vi "READ NavX.vi"() -> (1 "Status":T3 {"OP Status" items=["INITIALIZING", "SELFTEST_IN_PROGRESS", "ERROR", "IMU_AUTOCAL_IN_PROGRESS", "NORMAL"]; "Calibration Status" items=["IMU_CAL_STATE_MASK"=3, "IMU_CAL_STATE_INPROGRESS"=0, "IMU_CAL_STATE_ACCUMULATE"=1, "IMU_CAL_STATE_COMPLETE"=2]}, 3 "YRPHfH":T7)   [LabVIEW 2020]
uses:
  <vilib>/Rock Robotics/WPI/ThirdParty/Sensors/navX/_TypeDefs/Flags/Z900_navX_Flags_HardwareRevTypeDef.ctl
  <vilib>/Rock Robotics/WPI/ThirdParty/Sensors/navX/_TypeDefs/Flags/Z900_navX_Flags_OmnimountConfigTypeDef.ctl
  <vilib>/Rock Robotics/WPI/ThirdParty/Sensors/navX/_TypeDefs/Flags/Z900_navX_Flags_OpStatusTypeDef.ctl
  <vilib>/Rock Robotics/WPI/ThirdParty/Sensors/navX/_TypeDefs/Flags/Z900_navX_Flags_CalibrationStatusTypeDef.ctl
  <vilib>/Rock Robotics/WPI/ThirdParty/Sensors/navX/_TypeDefs/FRIC_navX_DeviceNumbersTypeDef.ctl
  <vilib>/Rock Robotics/Network Tables/NT Write Number.vi
panel:
  out "Board Information":T6 {"Board"."Hardware Revision" items=["navX-MXP"=33, "navX-Micro"=40]; "Omnimount Config" items=["DEFAULT", "X_UP", "X_DOWN", "Y_UP", "Y_DOWN", "Z_UP", "Z_DOWN"]}
  in  "main ref":string="NavX"
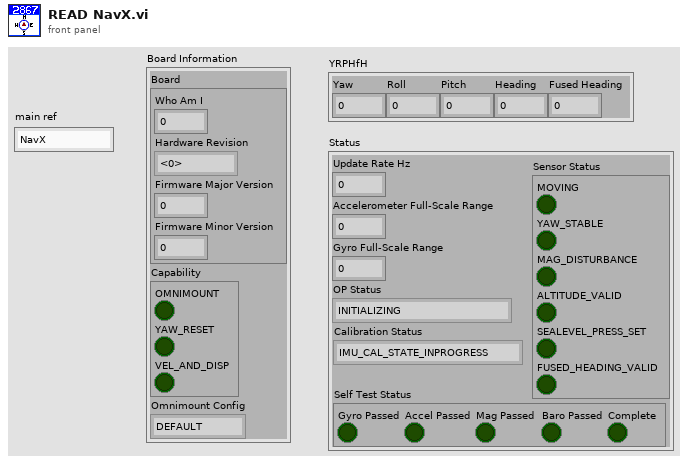
[diagram p1: front panel]
types:
  T1 = typedef "Z900_navX_Flags_OpStatusTypeDef.ctl" = u8
  T2 = typedef "Z900_navX_Flags_CalibrationStatusTypeDef.ctl" = u8
  T3 = cluster{"Update Rate Hz":u8, "Accelerometer Full-Scale Range":u8, "Gyro Full-Scale Range":u16, "OP Status":T1, "Calibration Status":T2, "Sensor Status":cluster{"MOVING":bool, "YAW_STABLE":bool, "MAG_DISTURBANCE":bool, "ALTITUDE_VALID":bool, "SEALEVEL_PRESS_SET":bool, "FUSED_HEADING_VALID":bool}, "Self Test Status":cluster{"Gyro Passed":bool, "Accel Passed":bool, "Mag Passed":bool, "Baro Passed":bool, "Complete":bool}}
  T4 = typedef "Z900_navX_Flags_HardwareRevTypeDef.ctl" = u8
  T5 = typedef "Z900_navX_Flags_OmnimountConfigTypeDef.ctl" = u8
  T6 = cluster{"Board":cluster{"Who Am I":u8, "Hardware Revision":T4, "Firmware Major Version":u8, "Firmware Minor Version":u8}, "Capability":cluster{"OMNIMOUNT":bool, "YAW_RESET":bool, "VEL_AND_DISP":bool}, "Omnimount Config":T5}
  T7 = cluster{"Yaw":dbl, "Roll":dbl, "Pitch":dbl, "Heading":dbl, "Fused Heading":dbl}
  T8 = typedef "FRIC_navX_DeviceNumbersTypeDef.ctl" = enum16{"Dev0", "Dev1", "Dev2", "Dev3"}
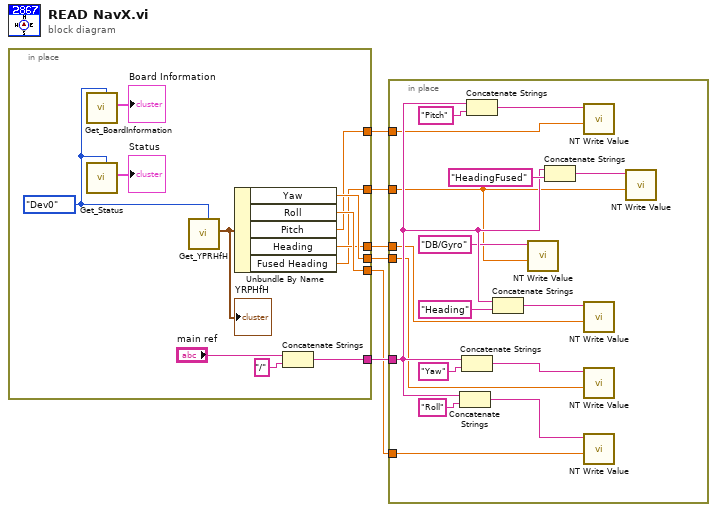
[diagram p0: block diagram]
diagram:
  n1 = in-place {
    in-place-border: [w15] -> w6
    in-place-border: [w14] -> w5
    in-place-border: [w13] -> w4
    in-place-border: [w12] -> w3
    in-place-border: [w11] -> w2
    in-place-border: [w10] -> w1
    w8 = FRIC_navX_DeviceNumbersTypeDef."Dev0" ("Device Number")
    n2 = call <vilib>:"Get_BoardInformation.vi"("Device Number"=w8) -> ("Board Information"=→"Board Information":T6)  [unwired: 10 in]
    n3 = call <vilib>:"Get_Status.vi"("Device Number"=w8) -> ("Status"=→"Status":T3)  [unwired: 10 in]
    n4 = call <vilib>:"Get_YPRHfH.vi"("Device Number"=w8) -> ("YRPHfH"=w16:T7)  [unwired: 10 in]
    "YRPHfH" <- w16
    n5 = Unbundle By Name(w16) -> ("Yaw"=w14:dbl, "Roll"=w13:dbl, "Pitch"=w12:dbl, "Heading"=w11:dbl, "Fused Heading"=w10:dbl)
    n6 = Concatenate Strings("main ref", "/" ("string")) -> (w15:string)
  }
  n7 = in-place {
    in-place-border: w6 -> [w25]
    in-place-border: w5 -> [w24]
    in-place-border: w4 -> [w23]
    in-place-border: w3 -> [w22]
    in-place-border: w2 -> [w21]
    in-place-border: w1 -> [w19]
    n8 = Concatenate Strings(w25, "Roll" ("string")) -> (w34:string)
    n9 = Concatenate Strings(w25, "Yaw" ("string")) -> (w35:string)
    n10 = Concatenate Strings(w25, "Pitch" ("string")) -> (w33:string)
    n11 = Concatenate Strings(w25, "Heading" ("string")) -> (w32:string)
    n12 = call-poly <vilib>:"NT Write Value.vi"("Numeric"=w19, "Name"="DB/Gyro") -> ()  [unwired: 9 in, 1 out]
    n13 = Concatenate Strings(w25, "HeadingFused" ("string")) -> (w27:string)
    n14 = call-poly <vilib>:"NT Write Value.vi"("Numeric"=w22, "Name"=w33) -> ()  [unwired: 9 in, 1 out]
    n15 = call-poly <vilib>:"NT Write Value.vi"("Numeric"=w21, "Name"=w32) -> ()  [unwired: 9 in, 1 out]
    n16 = call-poly <vilib>:"NT Write Value.vi"("Numeric"=w24, "Name"=w35) -> ()  [unwired: 9 in, 1 out]
    n17 = call-poly <vilib>:"NT Write Value.vi"("Numeric"=w23, "Name"=w34) -> ()  [unwired: 9 in, 1 out]
    n18 = call-poly <vilib>:"NT Write Value.vi"("Numeric"=w19, "Name"=w27) -> ()  [unwired: 9 in, 1 out]
  }
